vi "AFT Get Coefficients (FIR, Complex).vi"(8 "error in (no error)":errorcluster, 11 "adaptive filter in":refnum<k20>) -> (0 "error out":errorcluster, 2 "coefficients":cdb[](array[numeric]), 3 "adaptive filter out":refnum<k20>)   [LabVIEW 2017, in "NI_AdaptiveFilter.lvlib"]
doc: "Retrieves the filter coefficients from an adaptive filter that you create with the least mean squares (LMS) or recursive least squares (RLS) algorithms. You must manually select the polymorphic instance you want to use."
uses:
  <vilib>/addons/Adaptive Filters/NI_AdaptiveFilter.lvlib
  <resource>/AdaptiveFilters.dll
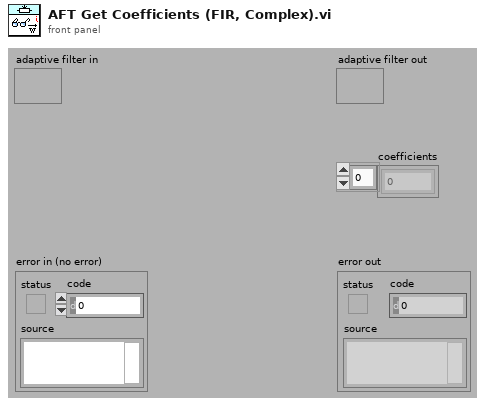
[diagram p1: front panel]
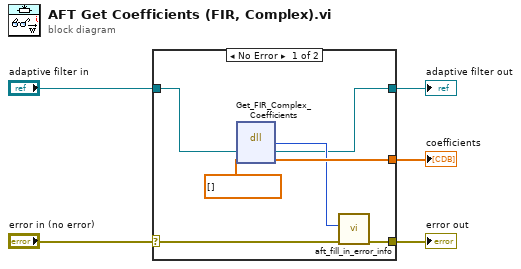
[diagram p0: block diagram]
diagram:
  n1 = case shown="No Error" "error in (no error)" {
    selector: "error in (no error)" -> [w12 w14]
    tunnel: [w11 w14] -> w5
    tunnel: "adaptive filter in" -> [w7 w13]
    tunnel: [w6 w13] -> w2
    tunnel: [w10 _] -> w4
    frame No Error {
      n2 = dll-call lib="C:/Program Files/National Instruments/LabVIEW 2017/resource/AdaptiveFilters.dll" fn="Get_FIR_Complex_Coefficients" ("Complex Data Initialization")("pSession"=w7, "Coeff"=cdb[] [] ("coefficients 2")) -> ("err"=w9:i32, "pSession"=w6:refnum<k20>, "Coeff"=w10:cdb[])  [unwired: 3 in, 2 out]
      n3 = call <vilib>:"aft_fill_in_error_info.vi"("error in"=w12, "status code"=w9) -> ("error out"=w11:errorcluster)  [unwired: 2 in, 7 out]
    }
    frame Error {
    }
  }
  "coefficients" <- w4
  "error out" <- w5
  "adaptive filter out" <- w2
